vi "Account For Texture Y Start.vi"(10 "Texture":T1, 11 "Point":T3) -> (3 "Point In Texture":T3)   [LabVIEW 2020, in "Raster (FPGA).lvlib"]
uses:
  Raster (FPGA).lvlib
  Point 2D (I32).ctl
  Texture.ctl
  Rectangle Dimensions.ctl
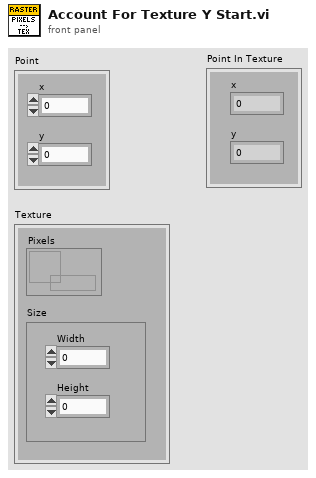
[diagram p1: front panel]
types:
  T1 = typedef "Raster (FPGA).lvlib/Texture.ctl" = cluster{"Pixels":refnum<data-value>, "Size":T2}
  T2 = typedef "Raster (FPGA).lvlib/Rectangle Dimensions.ctl" = cluster{"Width":u32, "Height":u32}
  T3 = typedef "Raster (FPGA).lvlib/Point 2D (I32).ctl" = cluster{"x":i32, "y":i32}
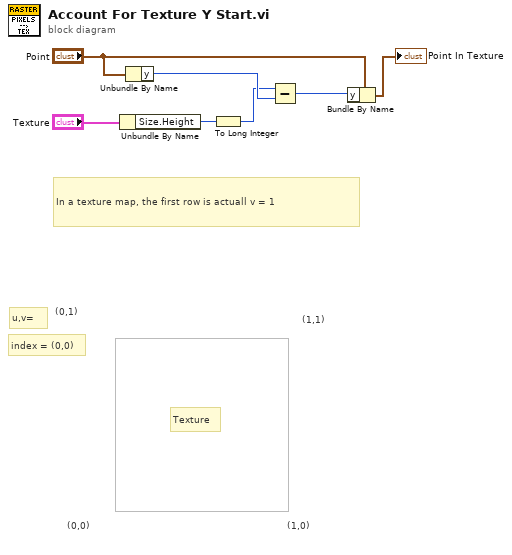
[diagram p0: block diagram]
diagram:
  # "index = (0,0)"
  # "u,v="
  # "Texture"
  # "(1,0)"
  # "(0,1)"
  # "(0,0)"
  # "(1,1)"
  # "In a texture map, the first row is actuall v = 1"
  n1 = Unbundle By Name("Texture") -> ("Size.Height"=w5:u32)
  n2 = Unbundle By Name("Point") -> ("y"=w4:i32)
  n3 = To Long Integer(number=w5) -> (32bit integer=w2:i32)
  n4 = Subtract(x=w2, y=w4) -> (x-y=w3:i32)
  n5 = Bundle By Name(cluster="Point", "y"=w3) -> (→"Point In Texture":T3)
